vi "fgv_lidars-img.vi"(7 "cmd":enum16{"create", "read", "close"}(ring), 8 "error in (no error)":errorcluster caption="error in") -> (3 "New Image":T1)   [LabVIEW 2019]
uses:
  <vilib>/vision/Image Controls.llb/IMAQ Image.ctl
panel:
  out "error out":errorcluster
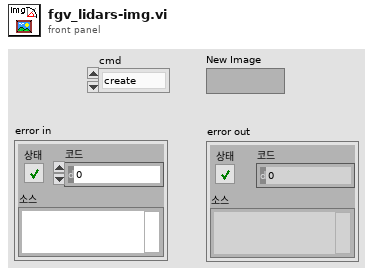
[diagram p1: front panel]
types:
  T1 = typedef "IMAQ Image.ctl" = refnum<image>
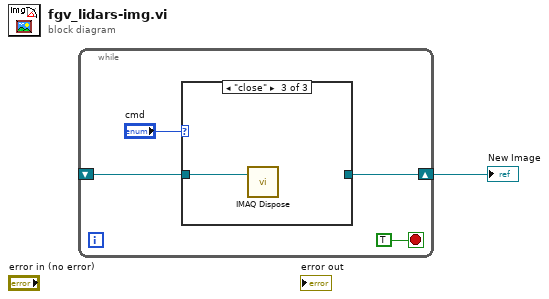
[diagram p0: block diagram]
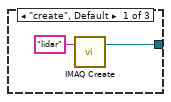
[diagram p2: hidden frame]
diagram:
  n1 = while {
    shift-right: [w3] -> w1
    shift-left: _ -> [w2]
    stop <- TRUE stop-if-true
    n2 = case shown="\"close\"" "cmd" {
      tunnel: [w6 w8 _] -> w3
      tunnel: w2 -> [_ w8 w9]
      frame "create", Default {
        n3 = call "IMAQ Create"("Image Name"="lidar") -> ("New Image"=w6:T1)  [unwired: 4 in, 1 out]
      }
      frame "read" {
      }
      frame "close" {
        n4 = call "IMAQ Dispose"("Image"=w9) -> ()  [unwired: 5 in, 1 out]
      }
    }
  }
  "New Image" <- w1
